vi "Example - Building an EXE.vi"() -> ()   [LabVIEW 2020]
doc: "Demonstrates the use of the Application Builder API to create and build an Application (EXE) build specification."
uses:
  <vilib>/AppBuilder/AB_API/common/AB_API Version Number.ctl
  <vilib>/AppBuilder/AB_API/EXE/NI_AB_API_EXE.lvclass
panel:
  in  "Enable debugging in EXE?":bool
  out "Generated Files":path[](array[path])
  # "Overview: Demonstrates the use of the Application Builder API to create and build an Application (EXE) build specification.\nRequirements: LabVIEW Professional Development System or LabVIEW Application Builder\nInstructions:\n1. Run the VI. An Application (EXE) build specification will be created, which will then be built programmatically.\n2. Examine the EXE build specification in the new project.\n3. Close the temporary project and delete the temporary project files generated by this example when you are done."
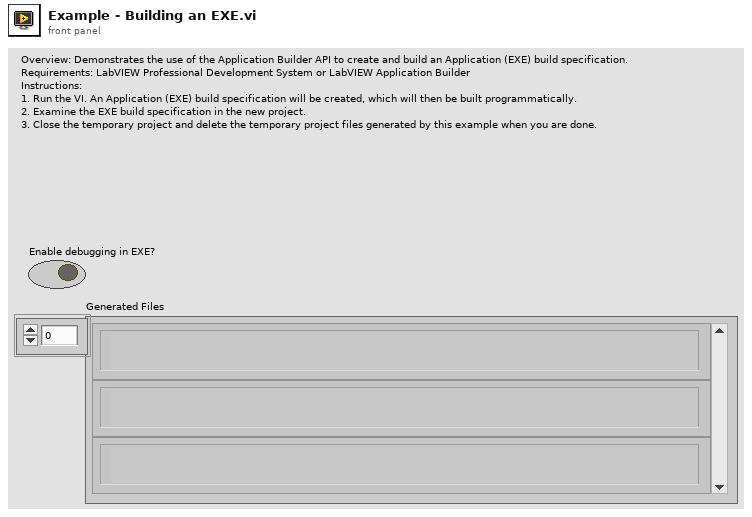
[diagram p1: front panel]
types:
  T1 = typedef "AB_API Version Number.ctl" = cluster{"Major":u16, "Minor":u16, "Fix":u16, "Build":u16}
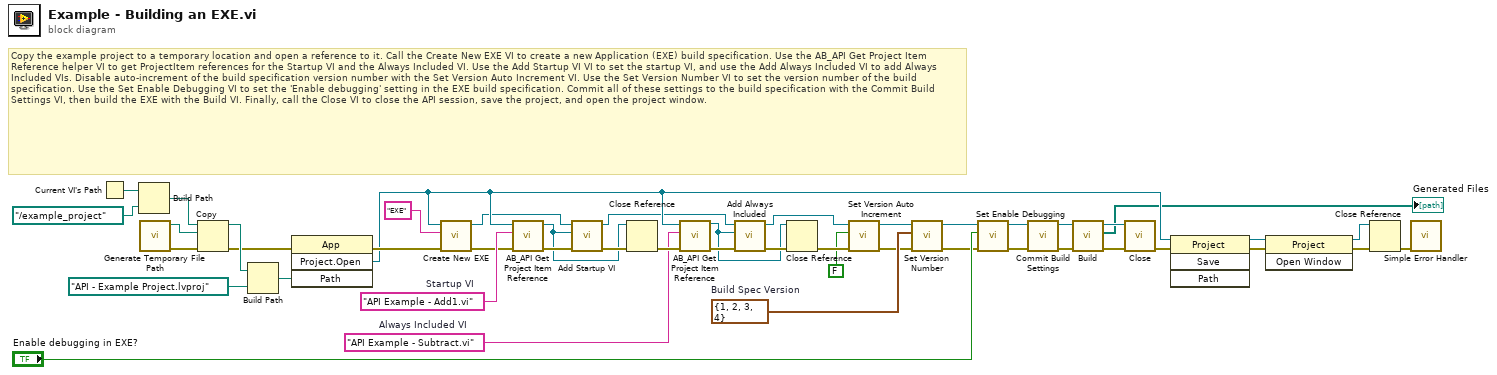
[diagram p0: block diagram]
diagram:
  w8 = T1 {"Major"=1, "Minor"=2, "Fix"=3, "Build"=4}  # Build Spec Version
  w24 = "API Example - Subtract.vi"  # Always Included VI
  w27 = "API Example - Add1.vi"  # Startup VI
  # "Copy the example project to a temporary location and open a reference to it. Call the Create New EXE VI to create a new Application (EXE) build specification. Use the AB_API Get Project Item Reference helper VI to get ProjectItem references for the Startup VI and the Always Included VI. Use the Add Startup VI VI to set the startup VI, and use the Add Always Included VI to add Always Included VIs. Disable auto-increment of the build specification version number with the Set Version Auto Increment VI. Use the Set Version Number VI to set the version number of the build specification. Use the Set Enable Debugging VI to set the 'Enable debugging' setting in the EXE build specification. Commit all of these settings to the build specification with the Commit Build Settings VI, then build the EXE with the Build VI. Finally, call the Close VI to close the API session, save the project, and open the project window."
  n1 = Current VI's Path() -> (path=w45:path)
  n2 = Build Path(base path=w45, name or relative path=path "../example_project" ("path")) -> (appended path=w42:path)
  n3 = call <vilib>:"Generate Temporary File Path.vi"() -> ("error out"=w35:errorcluster, "Unique Temporary File Path"=w41:path)  [unwired: 10 in]
  n4 = Copy(8:w35, 10:w41, 11:w42) -> (0:w34:errorcluster, 3:w40:path)  [unwired: 2 in, 1 out]
  n5 = Build Path(base path=w40, name or relative path=path "API - Example Project.lvproj") -> (appended path=w38:path)
  n6 = invoke class="App" method="Project.Open"(error in=w34, "Path"=w38) -> (error out=w44:errorcluster, "Project:Open"=w37:refnum<vi>)  [unwired: 2 in, 2 out]
  n7 = call <vilib>:"Create New EXE.vi"("error in (no error)"=w44, "Build specification name"="EXE", "Project Refnum"=w37) -> ("error out"=w23:errorcluster, "EXE out"=w18:refnum<class "NI_AB_API_EXE.lvclass">)  [unwired: 7 in]
  n8 = call <vilib>:"AB_API Get Project Item Reference.vi"("error in (no error)"=w23, "Name"=w27, "Project Refnum"=w37) -> ("error out"=w21:errorcluster, "ProjectItem Refnum"=w19:refnum<vi>)  [unwired: 6 in, 1 out]
  n9 = call-dynamic "Add Startup VI.vi"("error in (no error)"=w21, "ProjectItem Refnum"=w19, "EXE in"=w18) -> ("error out"=w20:errorcluster, "EXE out"=w15:refnum<class "NI_AB_API_EXE.lvclass">)  [unwired: 7 in]
  n10 = Close Reference(reference=w19, error in (no error)=w20) -> (error out=w26:errorcluster)
  n11 = call <vilib>:"AB_API Get Project Item Reference.vi"("error in (no error)"=w26, "Name"=w24, "Project Refnum"=w37) -> ("error out"=w17:errorcluster, "ProjectItem Refnum"=w14:refnum<vi>)  [unwired: 6 in, 1 out]
  n12 = call-dynamic "Add Always Included.vi"("error in (no error)"=w17, "ProjectItem Refnum"=w14, "EXE in"=w15) -> ("error out"=w16:errorcluster, "EXE out"=w6:refnum<class "NI_AB_API_EXE.lvclass">)  [unwired: 7 in]
  n13 = Close Reference(reference=w14, error in (no error)=w16) -> (error out=w25:errorcluster)
  n14 = call-dynamic "Set Version Auto Increment.vi"("error in (no error)"=w25, "Auto Increment Version"=FALSE, "NI_AB_API_EXE in"=w6) -> ("error out"=w7:errorcluster, "NI_AB_API_EXE out"=w5:refnum<class "NI_AB_API_EXE.lvclass">)  [unwired: 7 in]
  n15 = call-dynamic "Set Version Number.vi"("error in (no error)"=w7, "Version number"=w8, "EXE in"=w5) -> ("error out"=w10:errorcluster, "EXE out"=w9:refnum<class "NI_AB_API_EXE.lvclass">)  [unwired: 7 in]
  n16 = call-dynamic "Set Enable Debugging.vi"("error in (no error)"=w10, "Enable debugging (false)"="Enable debugging in EXE?", "EXE in"=w9) -> ("error out"=w13:errorcluster, "EXE out"=w12:refnum<class "NI_AB_API_EXE.lvclass">)  [unwired: 7 in]
  n17 = call-dynamic "Commit Build Settings.vi"("error in (no error)"=w13, "EXE in"=w12) -> ("error out"=w33:errorcluster, "EXE out"=w31:refnum<class "NI_AB_API_EXE.lvclass">)  [unwired: 8 in]
  n18 = call-dynamic "Build.vi"("error in (no error)"=w33, "EXE in"=w31) -> ("error out"=w32:errorcluster, "GeneratedFiles"=→"Generated Files":path[], "EXE out"=w30:refnum<class "NI_AB_API_EXE.lvclass">)  [unwired: 6 in, 1 out]
  n19 = call-dynamic "Close.vi"("error in (no error)"=w32, "EXE in"=w30) -> ("error out"=w29:errorcluster)  [unwired: 9 in]
  n20 = invoke class="Project" method="Save"(reference=w37, error in=w29) -> (reference out=w2:refnum<vi>, error out=w46:errorcluster)  [unwired: 2 in, 2 out]
  n21 = invoke class="Project" method="Open Window"(reference=w2, error in=w46) -> (reference out=w1:refnum<vi>, error out=w3:errorcluster)  [unwired: 1 in, 1 out]
  n22 = Close Reference(reference=w1, error in (no error)=w3) -> (error out=w43:errorcluster)
  n23 = call <vilib>:"Simple Error Handler.vi"("error in (no error)"=w43) -> ()  [unwired: 4 in, 5 out]
